vi "Swap 2nPort.vi"(8 "error in (no error)":errorcluster, 11 "Parameters In (2D)":cdb[][](array[numeric])) -> (0 "error out":errorcluster, 3 "Parameters Out (2D)":cdb[][](array[numeric]))   [LabVIEW 2023, in "NI_HFNetworkAnalysis.lvlib"]
doc: "Swap the ports of a 2n-Port network.\n\nThe last n ports become the input ports and the fisrt n ports become the output ports."
uses:
  NI_HFNetworkAnalysis.lvlib
  <vilib>/Analysis/Matrix/Numeric/Conversions/Array To Matrix - CA2.vi
  <vilib>/Analysis/Matrix/Numeric/Conversions/Matrix To Array - CM.vi
  <vilib>/Analysis/Matrix/NI_Matrix.lvlib
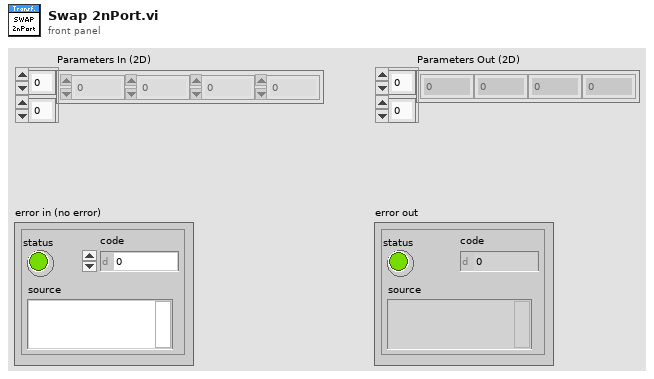
[diagram p1: front panel]
types:
  T1 = typedef "NI_Matrix.lvlib/ComplexMatrix.ctl" = cdb[][]
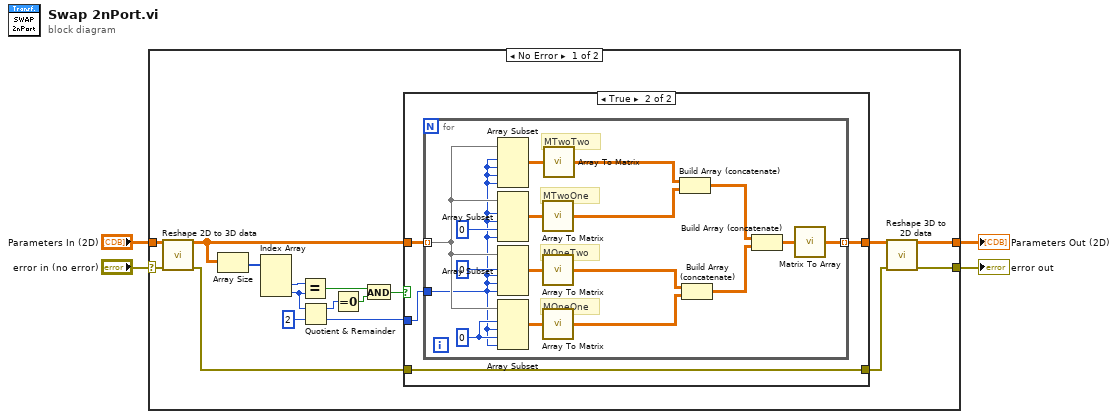
[diagram p0: block diagram]
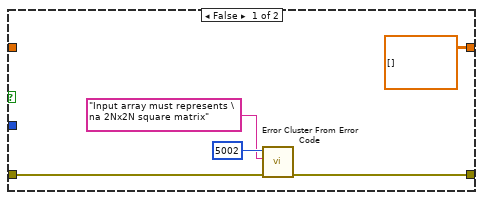
[diagram p2: hidden frame]
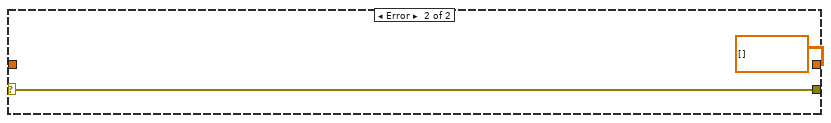
[diagram p3: hidden frame]
diagram:
  n1 = case shown="No Error" "error in (no error)" {
    selector: "error in (no error)" -> [w19 w49]
    tunnel: [w18 w49] -> w4
    tunnel: "Parameters In (2D)" -> [w21 _]
    tunnel: [w20 cdb[][] [] ("Array in")] -> w1
    frame No Error {
      n2 = call "Reshape 2D to 3D data.vi"("Parameters In (2D)"=w21, "Error In"=w19) -> ("Parameters Out (3D)"=w9:cdb[][][], "Error Out"=w6:errorcluster)  [unwired: 12 in]
      n3 = Array Size(array=w9) -> (size(s)=w17:i32[])
      n4 = Index Array(array=w17) -> (element #2=w12:i32, element #3=w16:i32)  [unwired: 3 in, 1 out]
      n5 = Equal?(x=w12, y=w16) -> (x = y?=w14:bool)
      n6 = Quotient & Remainder(x=w16, y=2) -> (x-y*floor(x/y)=w11:i32, floor(x/y)=w8:i32)
      n7 = Equal To 0?(x=w11) -> (x = 0?=w13:bool)
      n8 = And(x=w14, y=w13) -> (x .and. y?=w10:bool)
      n9 = case shown="True" w10 {
        tunnel: w9 -> [_ w30]
        tunnel: w8 -> [_ w29]
        tunnel: [cdb[][][] [] ("Complex 2D Array") w28] -> w7
        tunnel: w6 -> [w24 w27]
        tunnel: [w23 w27] -> w5
        frame False {
          n10 = call <vilib>:"Error Cluster From Error Code.vi"("error in (no error)"=w24, "error message (\"\")"="Input array must represents \na 2Nx2N square matrix" ("error message (\"\")"), "error code (0)"=5002) -> ("error out"=w23:errorcluster)  [unwired: 6 in]
        }
        frame True {
          n11 = for {
            tunnel: w30 -> [w40] mode=indexing
            tunnel: w29 -> [w39]
            tunnel: [w31] -> w28 mode=indexing
            w47 = 0 ("index")
            # "MTwoTwo"
            # "MTwoOne"
            # "MOneTwo"
            # "MOneOne"
            n12 = Array Subset(array=w40, index (row)=w39, length (row)=w39, index (col)=w39, length (col)=w39) -> (w41:cdb[][])
            n13 = Array Subset(array=w40, index (row)=w39, length (row)=w39, index (col)=0 ("index"), length (col)=w39) -> (w42:cdb[][])
            n14 = Array Subset(array=w40, index (row)=0 ("index"), length (row)=w39, index (col)=w39, length (col)=w39) -> (w43:cdb[][])
            n15 = Array Subset(array=w40, index (row)=w47, length (row)=w39, index (col)=w47, length (col)=w39) -> (w44:cdb[][])
            n16 = call-poly <vilib>:"Array To Matrix.vi"("Complex 2D Array"=w42) -> ("Complex Matrix"=w37:T1)
            n17 = call-poly <vilib>:"Array To Matrix.vi"("Complex 2D Array"=w43) -> ("Complex Matrix"=w36:T1)
            n18 = call-poly <vilib>:"Array To Matrix.vi"("Complex 2D Array"=w44) -> ("Complex Matrix"=w35:T1)
            n19 = call-poly <vilib>:"Array To Matrix.vi"("Complex 2D Array"=w41) -> ("Complex Matrix"=w38:T1)
            n20 = Build Array (concatenate)(w38, w37) -> (w34:T1)
            n21 = Build Array (concatenate)(w36, w35) -> (w33:T1)
            n22 = Build Array (concatenate)(w34, w33) -> (w32:T1)
            n23 = call-poly <vilib>:"Matrix To Array.vi"("Complex Matrix"=w32) -> ("Complex 2D Array"=w31:cdb[][])
          }
        }
      }
      n24 = call "Reshape 3D to 2D data.vi"("Parameters In (3D)"=w7, "Error In"=w5) -> ("Parameters Out (2D)"=w20:cdb[][], "Error Out"=w18:errorcluster)  [unwired: 12 in]
    }
    frame Error {
    }
  }
  "Parameters Out (2D)" <- w1
  "error out" <- w4
